vi "Send Update Event.vi"(8 "error in (no error)":errorcluster, 11 "File Handler in":refnum<class "File Handler.lvclass">) -> (0 "error out":errorcluster, 3 "File Handler out":refnum<class "File Handler.lvclass">)   [LabVIEW 2018, in "GLog.lvlib" / "File Handler.lvclass"]
uses:
  File Handler.lvclass
  C:/Users/Colin/Documents/software_projects/labview/glog/src/api/extension/formatting_handler_interface/Formatting Handler.lvclass
  File Update Event.ctl
  extension/formatting_handler_interface/Formatting Handler.lvclass/Formatting Handler.ctl
  File Handler.lvclass/File Handler.ctl
  extension/formatting_handler_interface/Read Name.vi
panel:
  # "Connector Pane"
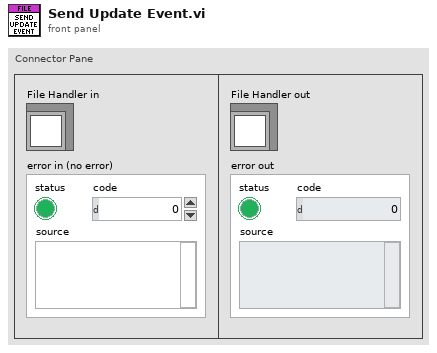
[diagram p1: front panel]
types:
  T1 = typedef "GLog.lvlib/File Handler.lvclass/File Update Event.ctl" = cluster{"Current File":path, "Source":string}
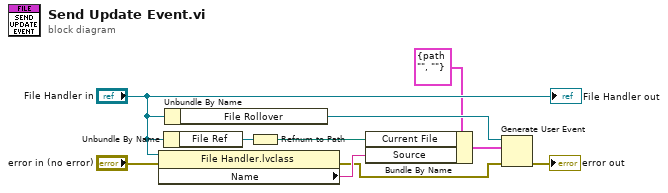
[diagram p0: block diagram]
diagram:
  n1 = property class="File Handler.lvclass"(reference="File Handler in", error in="error in (no error)") -> (error out=w1:errorcluster, "Name"=w5:string)  [unwired: 1 out]
  n2 = Unbundle By Name("File Handler in") -> ("File Ref"=w8:refnum<file>)
  n3 = Unbundle By Name("File Handler in") -> ("File Rollover"=w10:refnum<user-event>)
  n4 = Refnum to Path(1:w8) -> (0:w7:path)
  n5 = Bundle By Name(cluster=T1 {"Current File"=path "", "Source"=""} ("Rollover Event"), "Current File"=w7, "Source"=w5) -> (w3:T1)
  n6 = Generate User Event(user event=w10, event data cluster=w3, error in=w1) -> (error out=→"error out":errorcluster)  [unwired: 1 in, 1 out]
  "File Handler out" <- "File Handler in"
